vi "myRIO__TCP_connect_forReading.vi"(8 "input_error":errorcluster) -> (0 "output_error":errorcluster, 2 "output_connected":bool, 3 "output_hTCP":refnum<k5>)   [LabVIEW 2014]
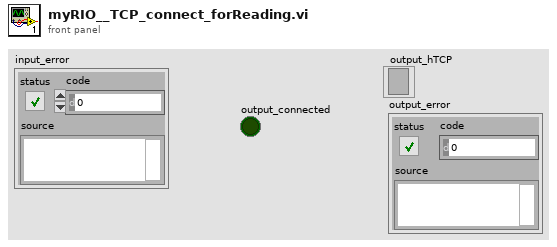
[diagram p1: front panel]
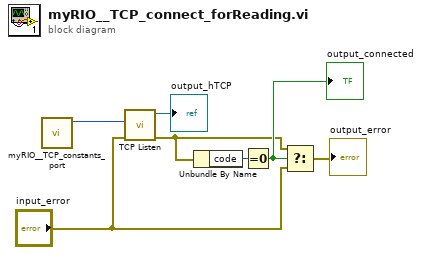
[diagram p0: block diagram]
diagram:
  n1 = call "myRIO__TCP_constants_port.vi"() -> ("output_TCP_port"=w1:u16)  [unwired: 11 in]
  n2 = call <vilib>:"TCP Listen.vi"("error in (no error)"="input_error", "port"=w1) -> ("error out"=w3:errorcluster, "connection ID"=→"output_hTCP":refnum<k5>)  [unwired: 5 in, 3 out]
  n3 = Unbundle By Name(w3) -> ("code"=w7:i32)
  n4 = Equal To 0?(x=w7) -> (x = 0?=w6:bool)
  "output_connected" <- w6
  n5 = Select(t=w3, s=w6, f="input_error") -> (s? t:f=→"output_error":errorcluster)
